vi "MPM_Get_System_Error.vi"(8 "error in (no error)":errorcluster, 11 ".NET Reference in":refnum<k24>) -> (0 "error out":errorcluster, 2 "error":string, 3 "Reference out":refnum<k24>)   [LabVIEW 2017]
uses:
  C:/Users/Ssantec_Test/Documents/Instrument_DLL_Sample_Labview_20250826_Ver1.5.0_x64/DLL/InstrumentDLL.dll
  DLL/InstrumentDLL.dll
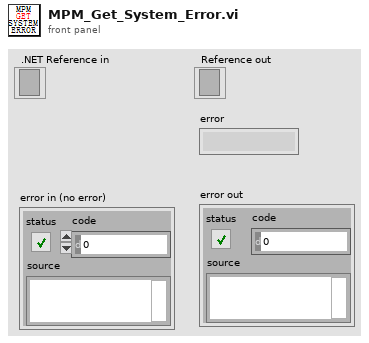
[diagram p1: front panel]
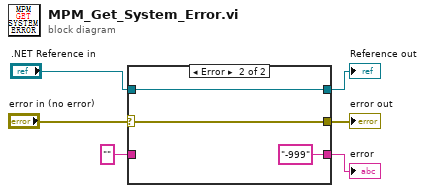
[diagram p0: block diagram]
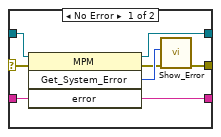
[diagram p2: hidden frame]
diagram:
  n1 = case shown="Error" "error in (no error)" {
    selector: "error in (no error)" -> [w7 w17]
    tunnel: [w14 "-999" ("error")] -> w6
    tunnel: ".NET Reference in" -> [w13 w15]
    tunnel: [w12 w15] -> w4
    tunnel: "" ("errorString") -> [w11 _]
    tunnel: [w8 w17] -> w2
    frame No Error {
      n2 = invoke on="调用节点" class="MPM" method="Get_System_Error"(reference=w13, error in=w7, "error"=w11) -> (reference out=w12:refnum<k24>, error out=w9:errorcluster, "Get_System_Error"=w10:i32, "error"=w14:string)  [unwired: 1 in]
      n3 = call "Show_Error.vi"("error in (no error)"=w9, "Error"=w10) -> ("error out"=w8:errorcluster)  [unwired: 9 in]
    }
    frame Error {
    }
  }
  "error" <- w6
  "Reference out" <- w4
  "error out" <- w2
